vi "PWM.Generate.Digital.vi"(11 "Settings":T1={"ACTIVE EDGE"=TRUE, "ACTIVE TICKS"=0, "INACTIVE TICKS"=0}) -> (3 "Output":bool)   [LabVIEW 2019, in "Speciality FPGA IO.lvlib"]
uses:
  Speciality FPGA IO.lvlib
  Types/PWM.Generate.Digital.Settings.ctl
  Types/PWM.Generate.Digital.Internal.ctl
panel:
  out "Local.Settings":T1
  out "Local.Data":T2
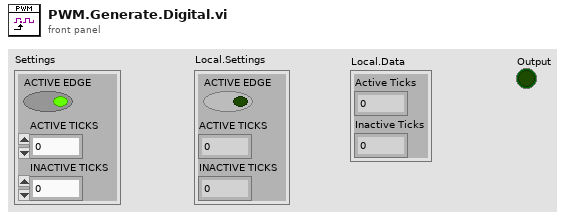
[diagram p1: front panel]
types:
  T1 = typedef "Speciality FPGA IO.lvlib/PWM.Generate.Digital.Settings.ctl" = cluster{"ACTIVE EDGE":bool, "ACTIVE TICKS":u32, "INACTIVE TICKS":u32}
  T2 = typedef "Speciality FPGA IO.lvlib/PWM.Generate.Digital.Internal.ctl" = cluster{"Active Ticks":u32, "Inactive Ticks":u32}
  T3 = enum8{"Initialize", "Active Edge", "Inactive Edge"}
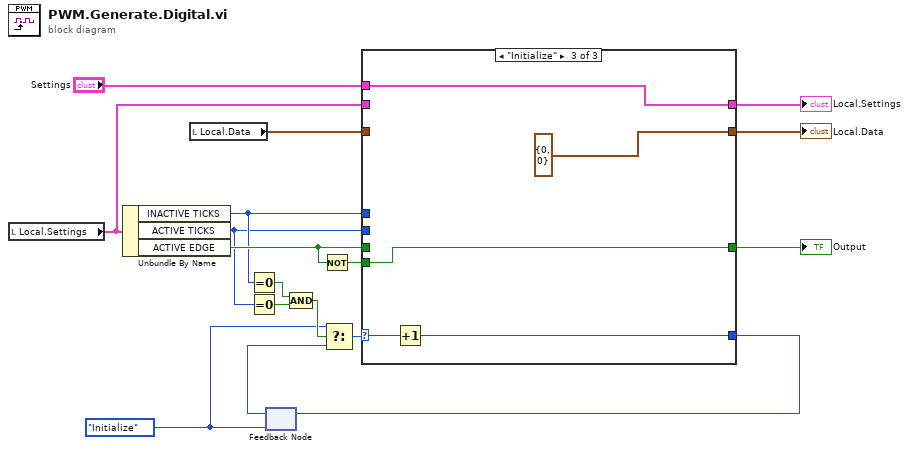
[diagram p0: block diagram]
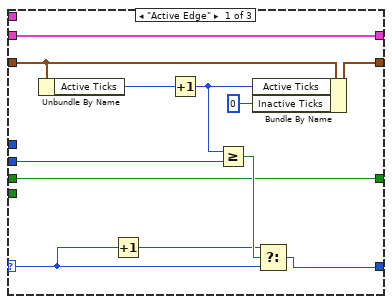
[diagram p2: hidden frame]
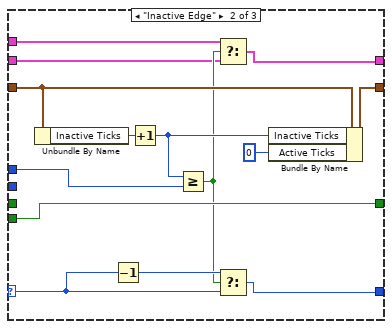
[diagram p3: hidden frame]
diagram:
  w4 = T3."Initialize"
  n1 = local read "Local.Settings"() -> (w9:T1)
  n2 = Unbundle By Name(w9) -> ("INACTIVE TICKS"=w8:u32, "ACTIVE TICKS"=w7:u32, "ACTIVE EDGE"=w13:bool)
  n3 = local read "Local.Data"() -> (w16:T2)
  n4 = Equal To 0?(x=w8) -> (x = 0?=w6:bool)
  n5 = Equal To 0?(x=w7) -> (x = 0?=w1:bool)
  n6 = feedback #1(w4) -> (w3:T3)
  n7 = Compound Arithmetic op=AND(w6, w1) -> (w5:bool)
  n8 = Not(x=w13) -> (.not. x?=w12:bool)
  n9 = Select(t=w4, s=w5, f=w3) -> (s? t:f=w2:T3)
  n10 = case shown="\"Initialize\"" w2 {
    selector: w2 -> [w19 w30 w48]
    tunnel: [w29 w43 T2 {"Active Ticks"=0, "Inactive Ticks"=0} ("Cached.Data")] -> w17
    tunnel: [w25 w40 w47] -> w14
    tunnel: w16 -> [w28 w42 _]
    tunnel: [w24 w35 w45] -> w15
    tunnel: w13 -> [w24 _ _]
    tunnel: w7 -> [w18 _ _]
    tunnel: w12 -> [_ w35 w45]
    tunnel: [w20 w32 w44] -> w11
    tunnel: "Settings" -> [_ w31 w44]
    tunnel: w8 -> [_ w36 _]
    tunnel: w9 -> [w20 w33 _]
    frame "Active Edge" {
      n11 = Unbundle By Name(w28) -> ("Active Ticks"=w27:u32)
      n12 = Increment(x=w19) -> (x+1=w21:T3)
      n13 = Increment(x=w27) -> (x+1=w23:u32)
      n14 = Greater Or Equal?(x=w23, y=w18) -> (x >= y?=w26:bool)
      n15 = Bundle By Name(cluster=w28, "Active Ticks"=w23, "Inactive Ticks"=u32 0) -> (w29:T2)
      n16 = Select(t=w21, s=w26, f=w19) -> (s? t:f=w25:T3)
    }
    frame "Inactive Edge" {
      n17 = Unbundle By Name(w42) -> ("Inactive Ticks"=w41:u32)
      n18 = Decrement(x=w30) -> (x-1=w37:T3)
      n19 = Increment(x=w41) -> (x+1=w39:u32)
      n20 = Greater Or Equal?(x=w39, y=w36) -> (x >= y?=w34:bool)
      n21 = Select(t=w31, s=w34, f=w33) -> (s? t:f=w32:T1)
      n22 = Select(t=w37, s=w34, f=w30) -> (s? t:f=w40:T3)
      n23 = Bundle By Name(cluster=w42, "Inactive Ticks"=w39, "Active Ticks"=u32 0 ("Inactive Ticks")) -> (w43:T2)
    }
    frame "Initialize" {
      n24 = Increment(x=w48) -> (x+1=w47:T3)
    }
  }
  "Local.Data" <- w17
  "Output" <- w15
  "Local.Settings" <- w11
  n25 = feedback-in #1(w14) -> ()
